vi "(SubVI)Waveform Editor_Build WF Seq.vi"(8 "error in (no error)":errorcluster caption="에러 입력(에러 없음)", 9 "Name (empty)":string, 10 "Sampling Rate":u32, 11 "WF Seq":refnum<class "Waveform Obj.lvclass">[](array[class])) -> (0 "error out":errorcluster caption="에러 출력", 1 "number of wf samples":i32, 2 "waveform out":waveform(i8), 3 "WF List Elements":T1, 4 "8bit memory data":u8[](array[numeric]), 6 "bytes of memory data":i32)   [LabVIEW 2020]
uses:
  Controls/(Ctrl)Waveform Editor_WF List.ctl
  Libraries/Waveform Obj Class/Waveform Obj/Waveform Obj.lvclass
  Libraries/Waveform Obj Class/Waveform Obj/Waveform Obj.lvclass/Waveform Obj.ctl
  Libraries/Waveform Obj Class/Waveform Obj/Accessors/Write sampling rate.vi
  Libraries/Waveform Obj Class/Waveform Obj/Accessors/Read voltage range.vi
  <vilib>/Waveform/WDTOps.llb/WDT Append Waveforms DBL.vi
  <vilib>/Waveform/WDTOps.llb/WDT Number of Waveform Samples DBL.vi
  <vilib>/Waveform/WDTOps.llb/WDT Waveform Duration DBL.vi
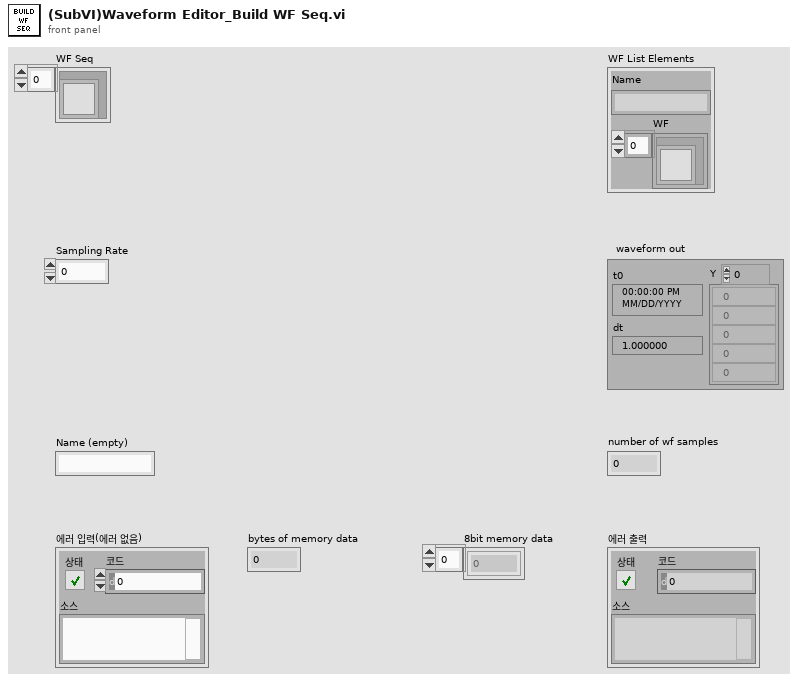
[diagram p1: front panel]
types:
  T1 = typedef "(Ctrl)Waveform Editor_WF List.ctl" = cluster{"Name":string, "WF Seq":refnum<class "Waveform Obj.lvclass">[]}
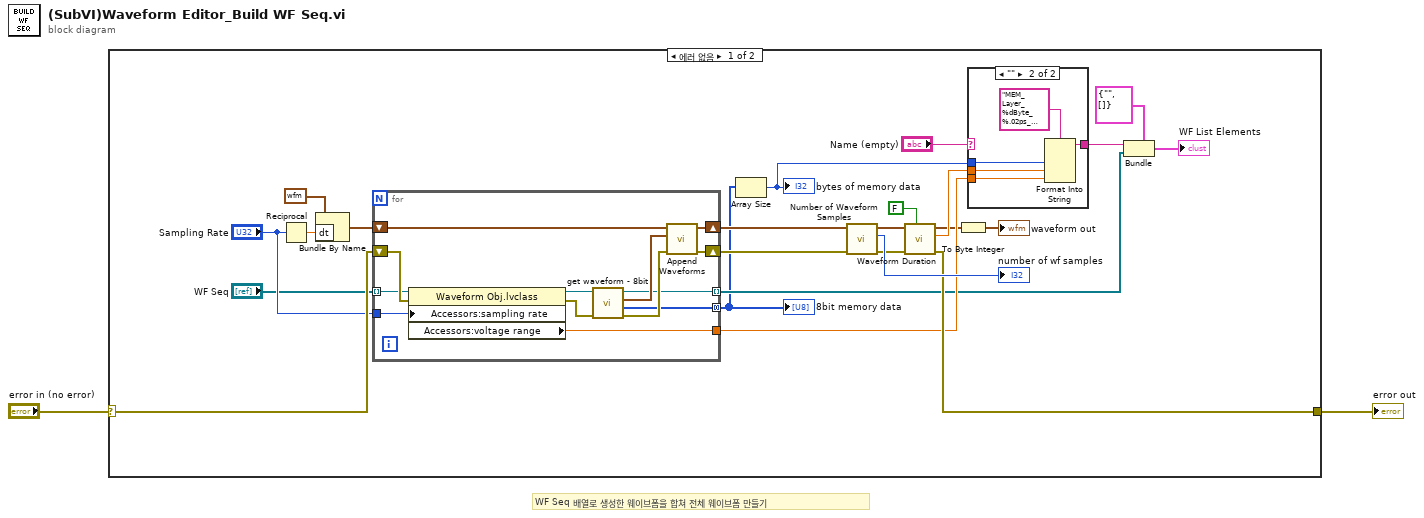
[diagram p0: block diagram]
diagram:
  # "WF Seq 배열로 생성한 웨이브폼을 합쳐 전체 웨이브폼 만들기"
  n1 = case shown="에러 없음" "error in (no error)" {
    selector: "error in (no error)" -> [w12 w46]
    tunnel: [w11 w46] -> w1
    frame No Error {
      n2 = Reciprocal(x="Sampling Rate") -> (1/x=w22:dbl)
      n3 = Bundle By Name(cluster=waveform(dbl) {"t0"=timestamp(0 s since 1904-01-01), "dt"=1.0, "Y"=[]} ("waveform A"), "dt"=w22) -> (w23:waveform(dbl))
      n4 = for {
        tunnel: "WF Seq" -> [w38] mode=indexing
        shift-right: [w43] -> w21
        shift-left: w23 -> [w44]
        shift-right: [w41] -> w14
        shift-left: w12 -> [w40]
        tunnel: "Sampling Rate" -> [w36]
        tunnel: [w35] -> w9
        tunnel: [w34] -> w6 mode=indexing
        tunnel: [w33] -> w4 mode=concatenating
        n5 = property class="Waveform Obj.lvclass"(reference=w38, error in=w40, "Accessors:sampling rate"=w36) -> (reference out=w37:refnum<class "Waveform Obj.lvclass">, error out=w39:errorcluster, "Accessors:voltage range"=w35:dbl)
        n6 = call-dynamic "get waveform - 8bit.vi"("error in (no error)"=w39, "Waveform Obj 입력"=w37) -> ("error out"=w42:errorcluster, "8bit memory data"=w33:u8[], "8bit waveform"=w45:waveform(i8), "Waveform Obj 출력"=w34:refnum<class "Waveform Obj.lvclass">)  [unwired: 6 in]
        n7 = call-poly <vilib>:"Append Waveforms.vi"("error in (no error)"=w42, "waveform B"=w45, "waveform A"=w44) -> ("error out"=w41:errorcluster, "waveform out"=w43:waveform(dbl))  [unwired: 7 in]
      }
      "8bit memory data" <- w4
      n8 = Array Size(array=w4) -> (size(s)=w3:i32)
      "bytes of memory data" <- w3
      n9 = call-poly <vilib>:"Number of Waveform Samples.vi"("error in (no error)"=w14, "waveform in"=w21) -> ("error out"=w13:errorcluster, "number of samples"=→"number of wf samples":i32, "waveform out"=w19:waveform(dbl))  [unwired: 7 in]
      n10 = call-poly <vilib>:"Waveform Duration.vi"("open interval? (T)"=FALSE, "error in (no error)"=w13, "waveform in"=w19) -> ("error out"=w11:errorcluster, "duration"=w17:dbl, "waveform out"=w8:waveform(dbl))  [unwired: 6 in]
      n11 = To Byte Integer(number=w8) -> (8bit integer=→"waveform out":waveform(i8))
      n12 = case shown="\"\"" "Name (empty)" {
        selector: "Name (empty)" -> [w27 _]
        tunnel: [w27 w32] -> w15
        tunnel: w17 -> [_ w31]
        tunnel: w3 -> [_ w30]
        tunnel: w9 -> [_ w28]
        frame Default {
        }
        frame "" {
          n13 = Format Into String(format string="MEM_Layer_%dByte_%.02ps_%.02pV" ("포맷 문자열"), w30, w31, w28) -> (resulting string=w32:string)  [unwired: 2 in, 1 out]
        }
      }
      n14 = Bundle(cluster=T1 {"Name"="", "WF Seq"=[]} ("WF List Elements"), "Name"=w15, "WF Seq"=w6) -> (→"WF List Elements":T1)
    }
    frame Error {
    }
  }
  "error out" <- w1
